vi "libssh2_channel_signal_ex.vi"(8 "error in (no error)":errorcluster, 10 "signal name":string, 11 "channel":T1) -> (0 "error out":errorcluster)   [LabVIEW 2013, in "libssh2.lvlib"]
doc: "Send a signal (without \"SIG\" prefix) to a process previously opened on the channel.\n\nSignals depend on the OS of the SSH server and may be ignored.\n\nFor example:\n\"TERM\" - terminate the process.\n\"IGN\" - ignore the signal (no-op).\n\"CORE\" - terminate the process and dump core.\n\"STOP\" - stop the process.\n\"CONT\" - continue the process if it is currently stopped."
uses:
  libssh2.lvlib
  Channel Refnum.ctl
  Not A Channel.vi
  <vilib>/Utility/error.llb/Error Cluster From Error Code.vi
  Global Settings.vi
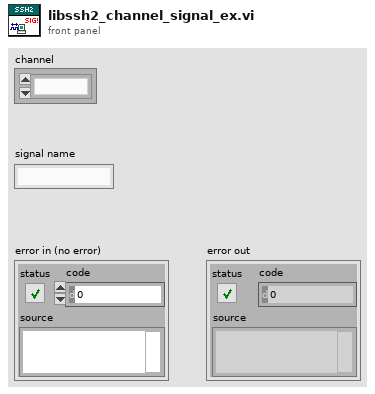
[diagram p1: front panel]
types:
  T1 = typedef "libssh2.lvlib/Channel Refnum.ctl" = refnum<k1>
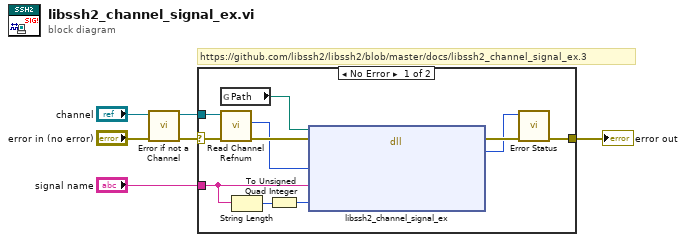
[diagram p0: block diagram]
diagram:
  # "https://github.com/libssh2/libssh2/blob/master/docs/libssh2_channel_signal_ex.3"
  n1 = call "Error if not a Channel.vi"("error in (no error)"="error in (no error)", "channel"="channel") -> ("error out"=w4:errorcluster, "channel out"=w2:T1)  [unwired: 8 in]
  n2 = case shown="No Error" w4 {
    selector: w4 -> [w17 w18]
    tunnel: [w16 w18] -> w6
    tunnel: w2 -> [w15 _]
    tunnel: "signal name" -> [w9 _]
    frame No Error {
      n3 = global read "Global Settings.vi" "Path"() -> (w11:path)
      n4 = call "Read Channel Refnum.vi"("error in (no error)"=w17, "channel"=w15) -> ("error out"=w13:errorcluster, "LIBSSH2_CHANNEL*"=w12:u64)  [unwired: 8 in]
      n5 = String Length(string=w9) -> (length=w8:i32)
      n6 = To Unsigned Quad Integer(1:w8) -> (0:w7:u64)
      n7 = dll-call lib="?" fn="libssh2_channel_signal_ex"(path in=w11, error in=w13, "channel"=w12, "signame"=w9, "signame_len"=w7) -> (error out=w14:errorcluster, "return value"=w10:i32)  [unwired: 4 in, 1 out]
      n8 = call "Error Status.vi"("error in (no error)"=w14, "return value"=w10) -> ("error out"=w16:errorcluster)  [unwired: 8 in, 1 out]
    }
    frame Error {
    }
  }
  "error out" <- w6
